vi "Tests_Window.vi"   [LabVIEW 2024]
uses:
  GLF/Window/Window.lvclass
  GLF/Engine/Engine.lvclass
  GLF/View/View.lvclass
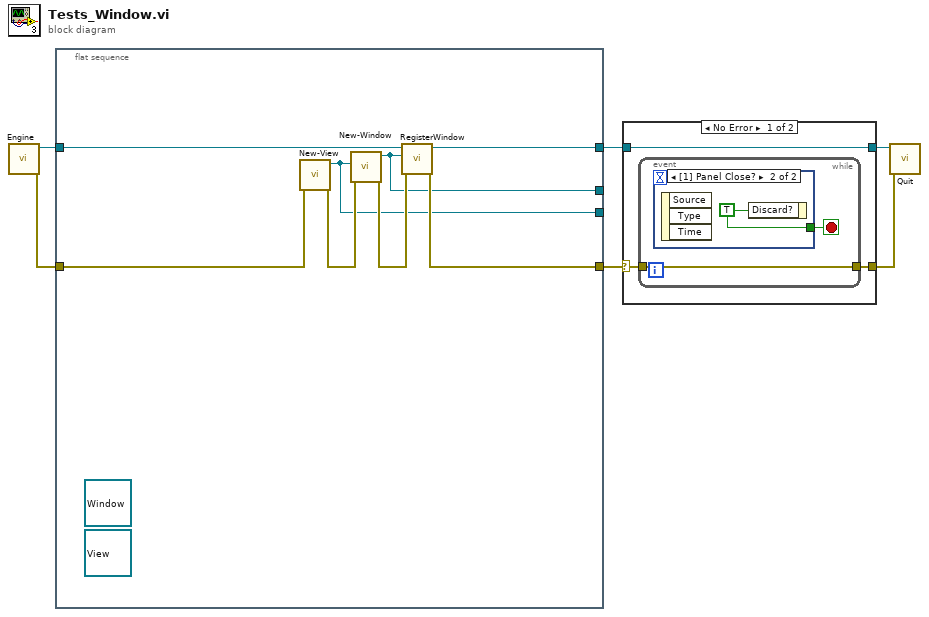
[diagram p0: block diagram]
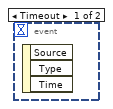
[diagram p2: hidden frame]
diagram:
  n1 = call "Engine.vi"() -> ("error out"=w5:errorcluster, "Engine"=w3:refnum<class "Engine.lvclass">)  [unwired: 10 in]
  n2 = flat-sequence {
    tunnel: w5 -> [w12]
    tunnel: [w9] -> w4
    tunnel: [w13] -> w1
    tunnel: w3 -> [w14]
    tunnel: [w8] -> _
    tunnel: [w7] -> _
    frame #0 {
      (unwired) refnum<class "View.lvclass"> refnum ("GLF.lvlib:View.lvclass")
      (unwired) refnum<class "Window.lvclass"> refnum ("GLF.lvlib:Window.lvclass")
      n3 = call "New-View.vi"("error in (no error)"=w12) -> ("error out"=w11:errorcluster, "View out"=w7:refnum<class "View.lvclass">)  [unwired: 9 in]
      n4 = call "New-Window.vi"("error in (no error)"=w11, "View"=w7) -> ("error out"=w10:errorcluster, "Window"=w8:refnum<class "Window.lvclass">)  [unwired: 8 in]
      n5 = call "RegisterWindow.vi"("error in (no error)"=w10, "Window"=w8, "Engine in"=w14) -> ("error out"=w9:errorcluster, "Engine out"=w13:refnum<class "Engine.lvclass">)  [unwired: 7 in]
    }
  }
  n6 = case shown="No Error" w4 {
    selector: w4 -> [w16 w21]
    tunnel: [w17 w21] -> w6
    tunnel: [w15 w22] -> w2
    tunnel: w1 -> [w15 w22]
    frame No Error {
      n7 = while {
        tunnel: w16 -> [w18]
        tunnel: [w18] -> w17
        stop <- w19 stop-if-true
        n8 = event shown="[1] Panel Close?" {
          selector: _ -> [_ _]
          dyn-events: _ -> [_ _]
          timeout: _ -> [_ _]
          tunnel: [_ w20] -> w19
          event Timeout {
            n9 = event-data() -> ()  [unwired: 1 in, 3 out]
          }
          event Panel Close? {
            w20 = TRUE ("Discard?")
            n10 = event-data() -> ()  [unwired: 1 in, 3 out]
            n11 = event-data("Discard?"=w20) -> ()  [unwired: 1 in, 1 out]
          }
        }
      }
    }
    frame Error {
    }
  }
  n12 = call "Quit.vi"("error in (no error)"=w6, "Engine in"=w2) -> ()  [unwired: 9 in, 1 out]
